vi "PM100-Read Power.vi"(0 "VISA in":refnum<visa-resource-name>, 7 "Duty cycle":dbl=1.0, 11 "error in (no error)":errorcluster) -> (4 "VISA out":refnum<visa-resource-name>, 6 "Readout String":string, 8 "Power (W)":dbl, 15 "error out":errorcluster)   [LabVIEW 2015]
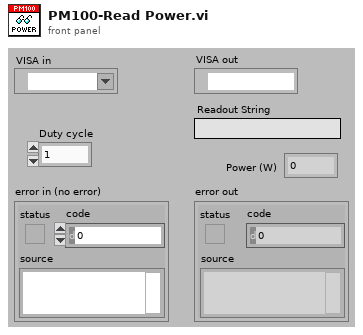
[diagram p1: front panel]
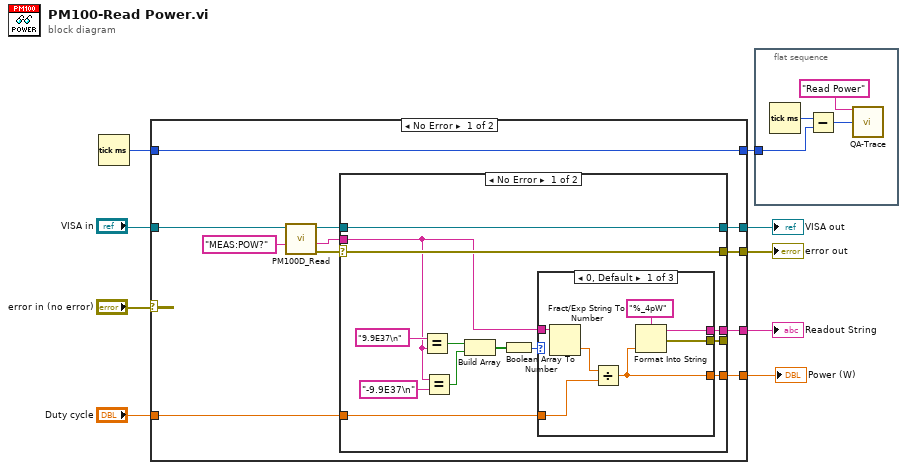
[diagram p0: block diagram]
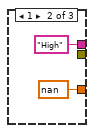
[diagram p2: hidden frame]
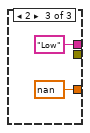
[diagram p3: hidden frame]
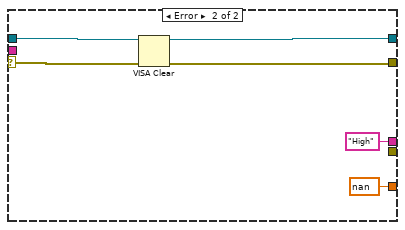
[diagram p4: hidden frame]
diagram:
  n1 = Tick Count (ms)() -> (millisecond timer value=w3:u32)
  n2 = case shown="No Error" "error in (no error)" {
    selector: "error in (no error)" -> [_ w52]
    tunnel: [w15 w52] -> w8
    tunnel: "VISA in" -> [w19 w51]
    tunnel: [w16 w51] -> w6
    tunnel: [w13 _] -> w5
    tunnel: [w12 _] -> w4
    tunnel: w3 -> [w11 _]
    tunnel: [w11 _] -> w2
    tunnel: "Duty cycle" -> [w10 _]
    frame No Error {
      n3 = call "PM100D_Read.vi"("Command"="MEAS:POW?", "VISA in"=w19) -> ("error out"=w18:errorcluster, "ReadValue"=w14:string, "VISA out"=w17:refnum<visa-resource-name>)  [unwired: 7 in]
      n4 = case shown="No Error" w18 {
        selector: w18 -> [w32 w48]
        tunnel: w17 -> [w33 w50]
        tunnel: [w33 w49] -> w16
        tunnel: [w32 w47] -> w15
        tunnel: w14 -> [w23 _]
        tunnel: [w30 "High"] -> w13
        tunnel: [w31 _] -> _
        tunnel: [w29 nan] -> w12
        tunnel: w10 -> [w21 _]
        frame No Error {
          n5 = Equal?(x="9.9E37\n", y=w23) -> (x = y?=w26:bool)
          n6 = Equal?(x=w23, y="-9.9E37\n") -> (x = y?=w25:bool)
          n7 = Build Array(w26, w25) -> (w28:bool[])
          n8 = Boolean Array To Number(Boolean array=w28) -> (number=w22:u32)
          n9 = case shown="0, Default" w22 {
            tunnel: [w40 _ _] -> w31
            tunnel: [w39 "High" "Low"] -> w30
            tunnel: w23 -> [w38 _ _]
            tunnel: [w36 nan nan] -> w29
            tunnel: w21 -> [w34 _ _]
            frame 0, Default {
              n10 = Fract/Exp String To Number(string=w38) -> (number=w35:dbl)  [unwired: 3 in, 1 out]
              n11 = Divide(x=w35, y=w34) -> (x/y=w36:dbl)
              n12 = Format Into String(format string="%_4pW", w36) -> (resulting string=w39:string, error out=w40:errorcluster)  [unwired: 2 in]
            }
            frame 1 {
            }
            frame 2 {
            }
          }
        }
        frame Error {
          n13 = VISA Clear(VISA resource name=w50, error in (no error)=w48) -> (VISA resource name out=w49:refnum<visa-resource-name>, error out=w47:errorcluster)
        }
      }
    }
    frame Error {
    }
  }
  "error out" <- w8
  "VISA out" <- w6
  "Readout String" <- w5
  "Power (W)" <- w4
  n14 = flat-sequence {
    tunnel: w2 -> [w55]
    frame #0 {
      n15 = Tick Count (ms)() -> (millisecond timer value=w56:u32)
      n16 = Subtract(x=w56, y=w55) -> (x-y=w54:u32)
      n17 = call "QA-Trace.vi"("trace string"="Read Power", "trace integer"=w54) -> ()  [unwired: 13 in, 1 out]
    }
  }
